vi "PvgeneratorOP500.vi"(8 "errin":errorcluster, 10 "network":path, 11 "path in":path) -> (0 "sortie d'erreur":errorcluster caption="errout", 1 "network out":path, 2 "tout bon":bool, 3 "Chaîne":string)   [LabVIEW 2020]
uses:
  VG/IS30%.vi
  VG/VG_OCV30min.vi
  VG/VG_OCV30max.vi
  VG/VG_OCV70min.vi
  VG/VG_OCV70max.vi
  VG/VG_OP400.vi
  VG/VG_ISOmin.vi
  VG/VG_DCIRmax.vi
  VG/VG_DCIRmin.vi
  VG/VG_DCIR+OUIouNON.vi
panel:
  out "nombre de remplacements":i32
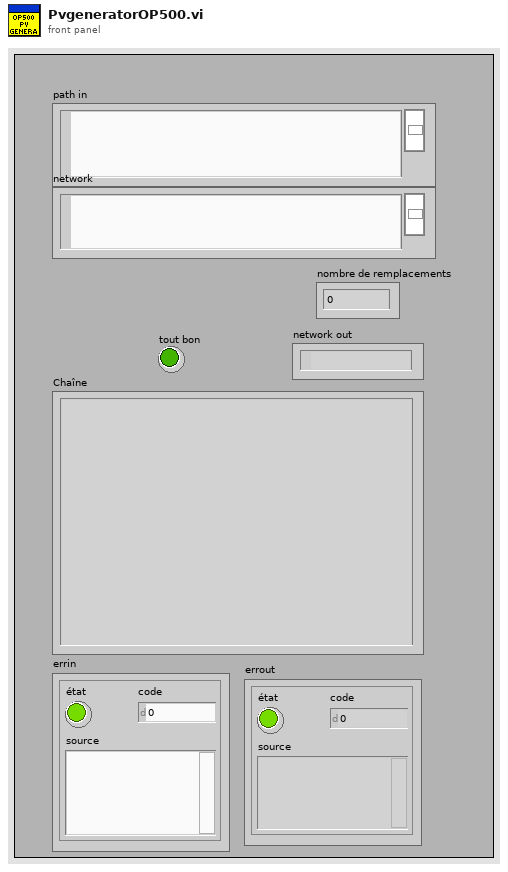
[diagram p1: front panel]
types:
  T1 = enum16{"open", "replace", "create", "open or create", "replace or create", "replace or create with confirmation"}
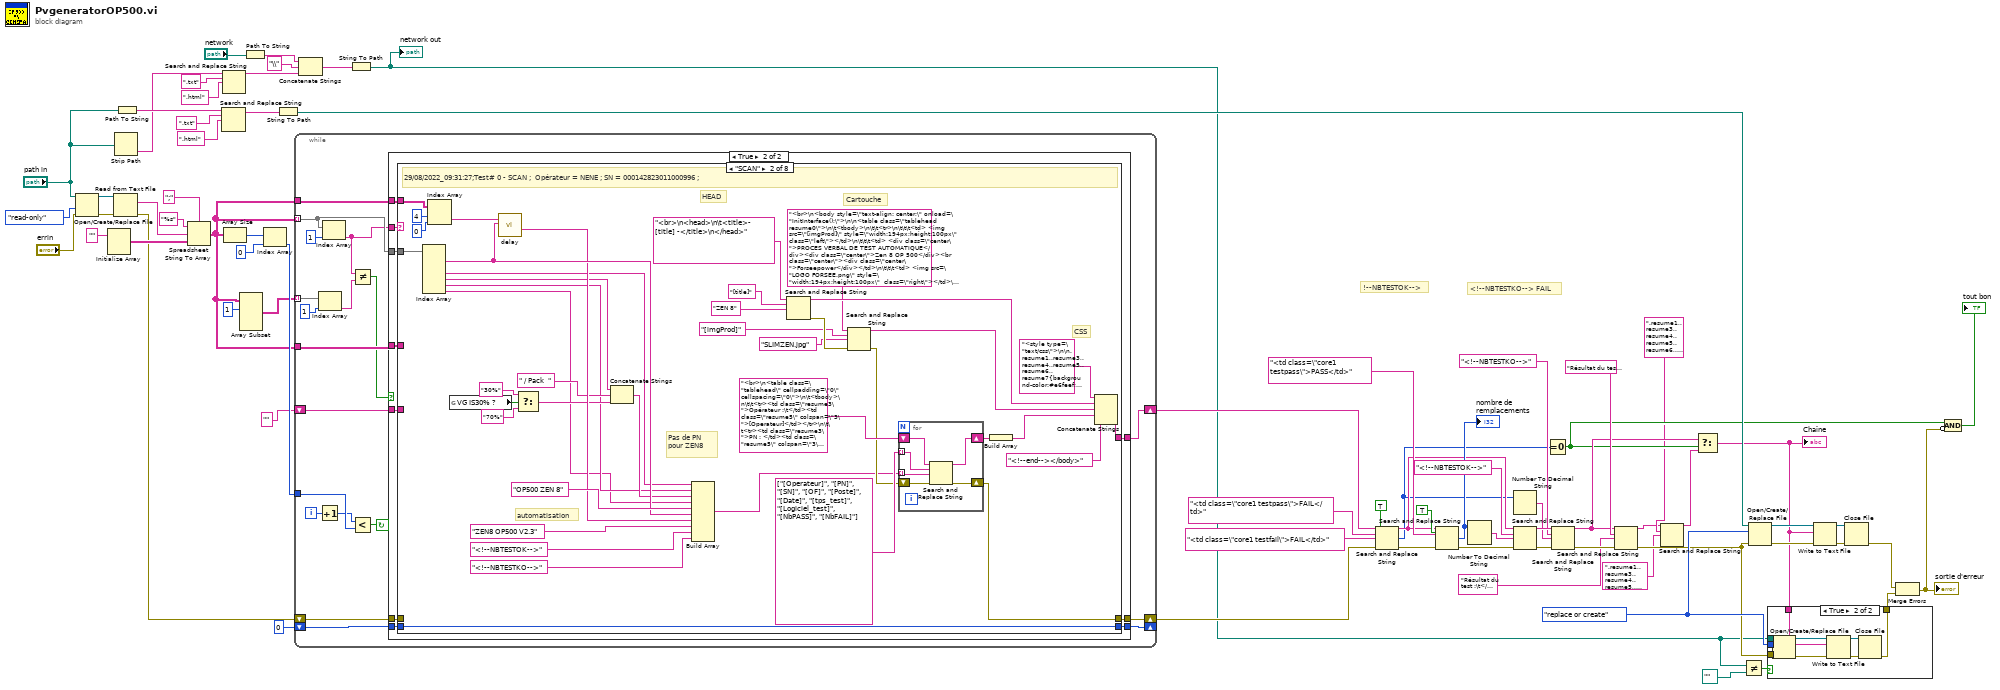
[diagram p0: block diagram]
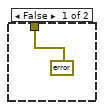
[diagram p2: hidden frame]
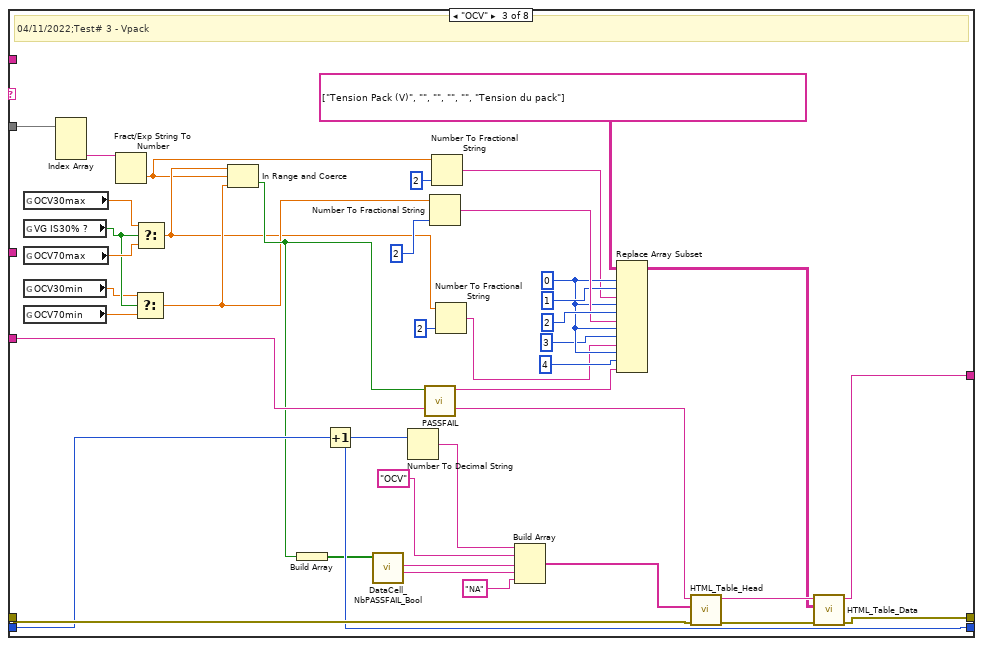
[diagram p5: hidden frame]
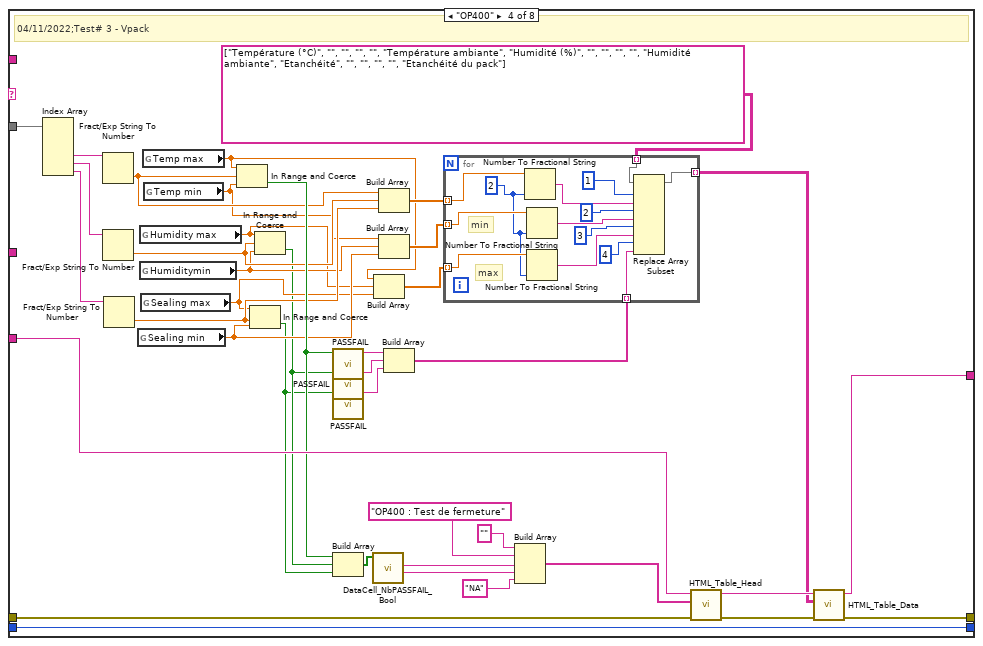
[diagram p6: hidden frame]
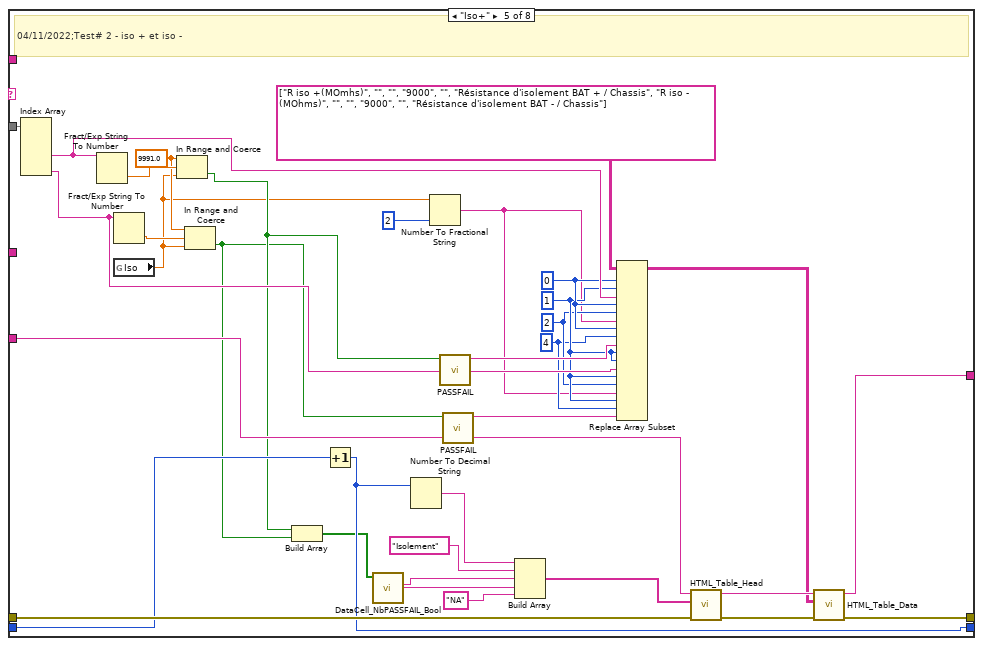
[diagram p7: hidden frame]
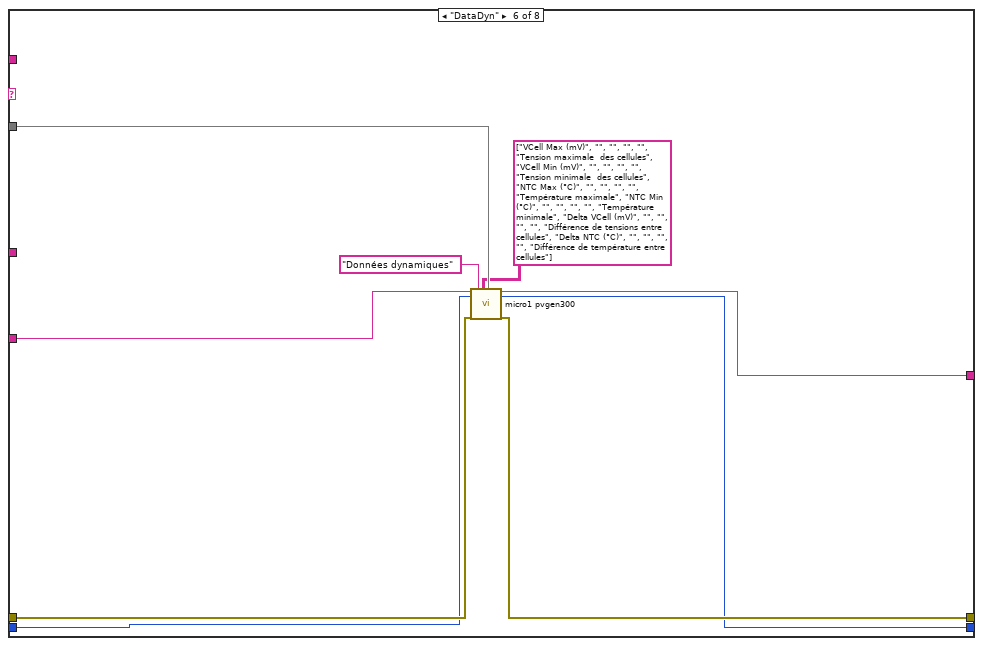
[diagram p8: hidden frame]
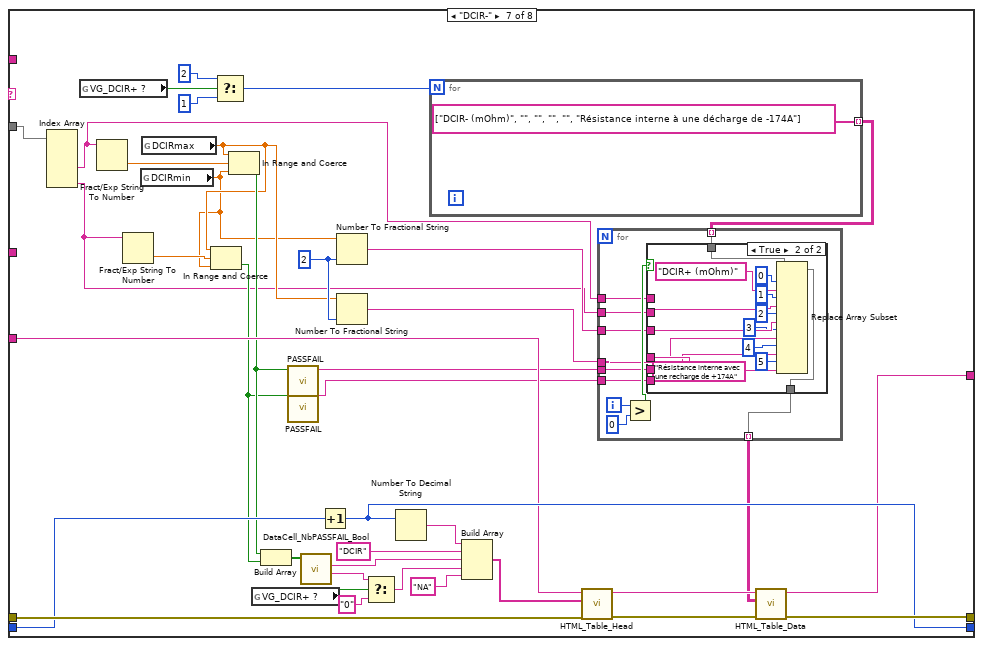
[diagram p9: hidden frame]
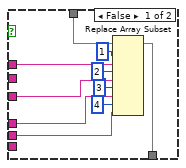
[diagram p10: hidden frame]
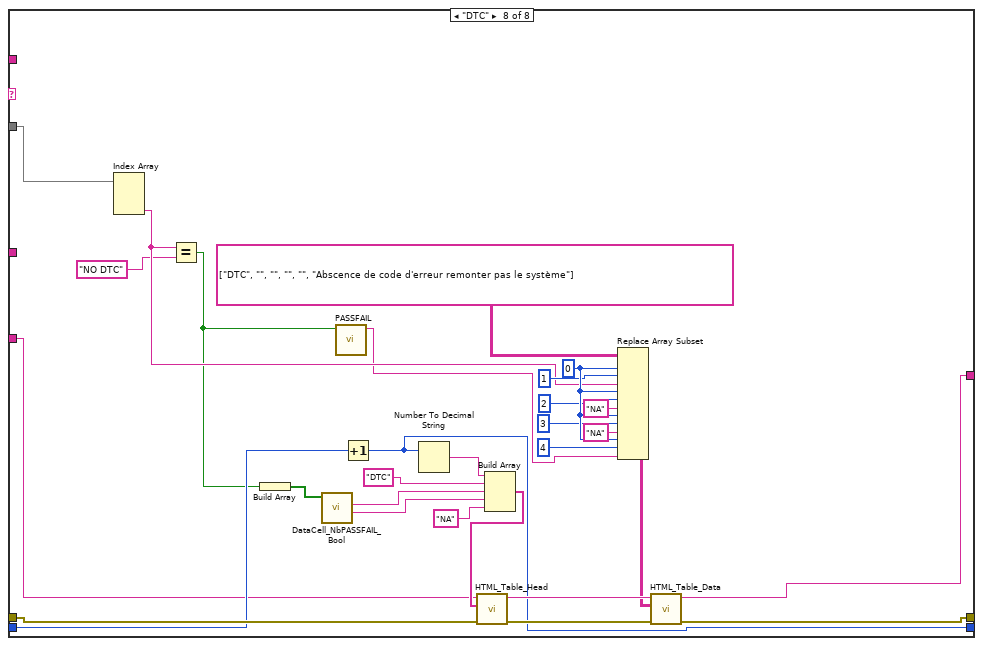
[diagram p11: hidden frame]
diagram:
  w32 = T1."replace or create" ("opération (0 : open)")
  # "<!--NBTESTKO--> FAIL"
  # "!--NBTESTOK-->"
  n1 = Open/Create/Replace File(file path (use dialog)="path in", error in="errin", access (0:read/write)=enum16{"read/write", "read-only", "write-only"}."read-only" ("accès (0 : read/write)")) -> (refnum out=w55:refnum<file>, error out=w72:errorcluster)  [unwired: 3 in, 1 out]
  n2 = Initialize Array("") -> (w70:string[][])  [unwired: 2 in]
  n3 = Read from Text File(file (use dialog)=w55, error in=w72) -> (text=w68:string, error out=w60:errorcluster)  [unwired: 2 in, 2 out]
  n4 = Strip Path(path="path in") -> (name=w13:string)  [unwired: 1 out]
  n5 = Path To String(path="path in") -> (string=w54:string)
  n6 = Spreadsheet String To Array(delimiter (Tab)=";" ("séparateur (Tabulation)"), format string="%s" ("chaîne de format"), spreadsheet string=w68, array type (2D Dbl)=w70) -> (array=w3:string[][])
  n7 = Search and Replace String(input string=w54, search string=".txt" ("chaîne recherchée"), replace string=".html" ("chaîne de remplacement (\"\")")) -> (result string=w51:string)  [unwired: 5 in, 3 out]
  n8 = Search and Replace String(input string=w13, search string=".txt" ("chaîne recherchée"), replace string=".html" ("chaîne de remplacement (\"\")")) -> (result string=w10:string)  [unwired: 5 in, 3 out]
  n9 = Array Size(array=w3) -> (size(s)=w66:i32[])
  n10 = Array Subset(array=w3, index (row)=1 ("indice")) -> (w1:string[][])  [unwired: 3 in]
  n11 = Path To String(path="network") -> (string=w12:string)
  n12 = Index Array(array=w66, index=0 ("indice")) -> (element=w64:i32)
  n13 = String To Path(string=w51) -> (path=w50:path)
  n14 = while {
    tunnel: w64 -> [w91]
    tunnel: w3 -> [w88] mode=indexing
    shift-right: [w87] -> w47
    shift-left: w60 -> [w86]
    shift-right: [w80] -> w49
    shift-left: "" -> [w85]
    shift-right: [w83] -> _
    shift-left: 0 -> [w84]
    tunnel: w3 -> [w82]
    tunnel: w3 -> [w79]
    tunnel: w1 -> [w77] mode=indexing
    i -> [w92]
    stop <- w90 continue-if-true
    n15 = Index Array(array=w77, index=1 ("indice")) -> (element=w76:string)
    n16 = Increment(x=w92) -> (x+1=w81:i32)
    n17 = Index Array(array=w88, index=1 ("indice")) -> (element=w75:string)
    n18 = Less?(x=w81, y=w91) -> (x < y?=w90:bool)
    n19 = Not Equal?(x=w75, y=w76) -> (x != y?=w74:bool)
    n20 = case shown="True" w74 {
      tunnel: w88 -> [_ w105]
      tunnel: [w94 w104] -> w87
      tunnel: w86 -> [w94 w103]
      tunnel: w85 -> [w95 w102]
      tunnel: w84 -> [w93 w101]
      tunnel: [w93 w100] -> w83
      tunnel: w82 -> [_ w99]
      tunnel: [w95 w98] -> w80
      tunnel: w75 -> [_ w97]
      tunnel: w79 -> [_ w96]
      frame False {
      }
      frame True {
        n21 = case shown="\"SCAN\"" w97 {
          tunnel: w103 -> [w108 _ w187 w227 w274 w291 w324 w391]
          tunnel: w105 -> [_ w149 w188 w228 w275 w287 w328 w381]
          tunnel: [w108 w128 w186 w226 w273 w290 w326 w392] -> w104
          tunnel: w102 -> [w106 _ w185 w225 w272 w285 w318 w382]
          tunnel: w101 -> [w107 w127 w184 w216 w271 w284 w323 w384]
          tunnel: [w107 w127 w183 w216 w270 w283 w320 w366] -> w100
          tunnel: w99 -> [_ _ _ _ _ _ _ _]
          tunnel: [w106 w126 w182 w224 w269 w289 w311 w380] -> w98
          tunnel: w96 -> [_ w125 _ _ _ _ _ _]
          frame "NULL", Default {
            # "NULL"
          }
          frame "SCAN" {
            # "automatisation"
            # "Pas de PN pour ZEN8"
            # "Cartouche"
            # "HEAD"
            # "CSS"
            # "29/08/2022_09:31:27;Test# 0 - SCAN ;  Opérateur = NENE ; SN = 000142823011000996 ;"
            n22 = Index Array(array=w149) -> (element #1=w121:string, element #3=w112:string, element #4=w111:string, element #5=w110:string, element #6=w109:string)  [unwired: 6 in, 1 out]
            n23 = Index Array(array=w125, index (row)=4, index (col)=0 ("disabled index (col)")) -> (element=w122:string)
            n24 = global read "IS30%.vi" "VG IS30% ?"() -> (w113:bool)
            n25 = call "delay.vi"("String"=w121, "String 2"=w122) -> ("Delay calculé"=w120:string)  [unwired: 9 in]
            n26 = Select(t="30%" ("y"), s=w113, f="70%" ("y")) -> (s? t:f=w116:string)
            n27 = Concatenate Strings(w111, " / Pack  " ("chaîne"), w116) -> (w118:string)
            n28 = Build Array(w112, w110, w118, w109, "OP500 ZEN 8" ("chaîne"), w121, w120, "ZEN8 OP500 V2.3" ("chaîne"), "<!--NBTESTOK-->" ("chaîne"), "<!--NBTESTKO-->" ("chaîne")) -> (w129:string[])
            n29 = Search and Replace String(input string="<br>\n<head>\n\t<title>- [title] -</title>\n</head>", search string="[title]" ("chaîne recherchée"), replace string="ZEN 8" ("Title")) -> (result string=w145:string, error out=w144:errorcluster)  [unwired: 5 in, 2 out]
            n30 = Search and Replace String(input string="<br>\n<body style=\"text-align: center;\" onload=\"InitInterface();\">\n\n<table class=\"tablehead resume0\">\n\t<tbody>\n\t\t<tr>\n\t\t\t<td> <img src=\"[imgProd]\" style=\"width:194px;height:100px\" class=\"left\"></td>\n\t\t\t<td> <div class=\"center\">PROCES VERBAL DE TEST AUTOMATIQUE</div><div class=\"center\">Zen 8 OP 500</div><br class=\"center\"><div class=\"center\">Forseepower</div></td>\n\t\t\t<td> <img src=\"LOGO FORSEE.png\" style=\"width:194px;height:100px\"  class=\"right\"></td>\n\t\t</tr>\n\t</tbody>\n</table>", search string="[imgProd]", replace string="SLIMZEN.jpg" ("imgProd"), error in=w144) -> (result string=w142:string, error out=w139:errorcluster)  [unwired: 4 in, 2 out]
            n31 = for {
              shift-right: [w154] -> w138
              shift-left: "<br>\n<table class=\"tablehead\" cellpadding=\"0\" cellspacing=\"0\">\n\t<tbody>\n\t\t<tr><td class=\"resume3\">Opérateur :\t</td><td class=\"resume5\" colspan=\"3\">[Operateur]</td></tr>\n\t\t<tr><td class=\"resume3\">PN : </td><td class=\"resume5\" colspan=\"3\">[PN]</td></tr>\n\t\t<tr><td class=\"resume3\">SN : </td><td class=\"resume5\" colspan=\"3\">[SN]</td></tr>\n\t\t<tr><td class=\"resume3\">OF : </td><td class=\"resume5\" colspan=\"3\">[OF]</td></tr>\n\t\t<tr><td class=\"resume3\">Poste : </td><td class=\"resume5\" colspan=\"3\">[Poste]</td></tr>\t\t\n\t\t<tr><td class=\"resume3\">Date du test : </td><td class=\"resume5\" colspan=\"3\">[Date]</td></tr>\n\t\t<tr><td class=\"resume3\">Temps de test : </td><td class=\"resume5\" colspan=\"3\">[tps_test]</td></tr>\n\t\t<tr><td class=\"resume3\">Logiciel de test :\t</td><td class=\"resume5\" colspan=\"3\">[Logiciel_test]</td></tr>\n\t\t<tr><td class=\"resume3\">Résultat du test :\t</td><td class=\"resume5\" colspan=\"3\"><div><span style=\"float:left\" id=\"result\"><font size = \"5pt\" color=\"green\"><b>CONFORME</b></font><b><font size = \"5pt\"> ( </font><font size = \"5pt\" color=\"green\">[NbPASS] PASS </font>  <font size = \"5pt\"> / </font><font size = \"5pt\" color=\"red\">[NbFAIL] FAIL</font> <font size = \"5pt\"> ) </font></b></span></div></td></tr>\n\t</tbody>\n</table>" -> [w155]
              tunnel: string[] ["[Operateur]", "[PN]", "[SN]", "[OF]", "[Poste]", "[Date]", "[tps_test]", "[Logiciel_test]", "[NbPASS]", "[NbFAIL]"] -> [w151] mode=indexing
              tunnel: w129 -> [w150] mode=indexing
              shift-right: [w152] -> w128
              shift-left: w139 -> [w153]
              n32 = Search and Replace String(input string=w155, search string=w151, replace string=w150, error in=w153) -> (result string=w154:string, error out=w152:errorcluster)  [unwired: 4 in, 2 out]
            }
            n33 = Build Array(w138) -> (w137:string[])
            n34 = Concatenate Strings("<style type=\"text/css\">\n\n.resume1,.resume3,.resume4,.resume5,.resume6,.resume7{background-color:#e6feef;padding:7px;border:1px solid black;}\n.resume0{border:1px solid black;background-color:#e6feef;font-weight: bold;padding:0px;text-align: center;}\n.resume1{width:350px;text-align:right;font-weight:bold;}\n.resume3{width:350px;text-align:right;border-top:0px solid black;font-weight:bold;}\n.resume4{border-left:0px solid black;width:290px;}\n.resume5{width:290px;border-left:0px solid black;border-top:0px solid black;}\n.resume6{border-left:0px solid black;width:60px;}\n.resume7{border-left:0px solid black;border-top:0px solid black;width:60px;}\n.title1{text-align: left;background-color:#e6f4fe;padding:10px;border:1px solid #101010;}\n.title2{width: 30px;text-align: center;background-color:#e6f4fe;padding:1px;border:1px solid #101010;border-left:0px solid black;font-weight: bold;}\n.title2 a:link{text-decoration:none;}\n.entete0,.entete1,.entete2,.time2{text-align: center;background-color:#feeec9;padding:7px;border:1px solid black;font-weight: bold;}\n.entete0{width:45px;border-right:0px solid black;}\n.entete1{width:505px;}\n.entete2{width:95px;border-right:0px solid black;}\n.time2{border-left:0px solid black;width:145px;font-size:11px;}\n.core0,.core1,.core2,.core3,.core4,.time{text-align: center;background-color:#fafed3;padding:7px;border:1px solid black;}\n.core0, .core1,.core3,.core4{width:95px;border-top:0px solid black;border-right:0px solid black;}\n.core0{width:45px;}\n.core2{border-top:0px solid black;width:505px;}\n.core3{width:200px;}\n.core4{width:300px;}\n.time{width:145px;border-top:0px solid black;border-left:0px solid black;font-size:11px;}\n.false .core0,.false .core1,.false .core2,.false .core3,.false .core4,.false .time{background-color:#f4f4f4;}\n.false .entete0,.false .entete1,.false .entete2,.false .time2{background-color:#dadada;}\n.false .title1,.false .title2,.false .resultentete .testpass,.false .resultentete .testfail,.false .resultentete .testtime{background-color:#c5cac9;color: blue;}\n.false .title2 a:link{text-decoration:none;color: blue;}\n.comment1,.comment2,.time3{width: 890px;background-color:#e9e8e9;padding:7px;border:1px solid black;border-top:0px solid black;text-align:left;}\n.comment2{border-right:0px solid black;width: 45px;text-align: center;}\n.time3{width: 145px;border-left:0px solid black;font-size:11px;}\n.fixe1{background: -moz-linear-gradient(center top , #101010 10%, #555555 80%) repeat scroll 0 0 transparent;background: -webkit-gradient(linear, left top, left bottom, from(#101010), to(#555555));border:2px solid orange;position : fixed;margin-top:20px;display:none;overflow-y:scroll;max-height:350px;text-shadow: 0px 0px 0 #333333;text-align:left;font-size:10px;padding:10px;margin-left:-162px;border-radius: 15px 15px 15px 15px;}\n.menufixe, .menufixelock{background: -moz-linear-gradient(center top , #101010 80%, transparent 20%) repeat scroll 0 0 transparent;background: -webkit-gradient(linear, left top, left bottom, from(#101010), color-stop(0.65, #101010), to(transparent)) repeat scroll 0 0 transparent;margin: -52px 0px 0px -9px;width:100%;position:fixed;height:55px;-moz-transition: margin 1s;-webkit-transition: margin 1s;}\n.menufixelock, .menufixe:hover{margin: -9px 0px 0px -9px;}\n.lockmenu, .separation,.separationmenu{text-align:center;background: -moz-linear-gradient(center top , #555555 10%, #111111 80%) repeat scroll 0 0 transparent;background: -webkit-gradient(linear, left top, left bottom, from(#555555), to(#111111));border: 1px solid white;border-radius: 10px 10px 10px 10px;box-shadow: 0 -1px 1px #555555 inset;color: #999999;font-weight: bold;width: 100px;padding: 2px;text-decoration: none;}\n.tablehead{width: 1000px;font-family: Verdana;font-size: 12px;margin-left: auto;margin-right: auto;}\n.tablenull{font-family: Verdana;font-size: 11px;margin-left: auto;margin-right: auto;}\n.separationmenu:hover div{display: inline;}\n.lockmenu:hover, .separation:hover,.separationmenu:hover{border: 1px solid orange;cursor:pointer;}\n.lockmenu:hover{border: 1px solid red;cursor:pointer;}\n.separationright{padding:10px;}\ndiv a:link{text-decoration:none;color:#cbcbcb;}\ndiv a:hover{text-decoration:underline;color:#cbcbcb;}\nspan a:link{text-decoration:none;color:#cbcbcb;}\nspan a:hover{text-decoration:none;color:#cbcbcb;}\n.false{color: blue;}\n.testpass{color: green;font-weight: bold;}\n.testfail{color: red;font-weight: bold;}\n.testtime{color: blue;font-weight: bold;}\n.resultentete{font-weight: bold;font-size: 11px;min-width: 200px;text-align:right;}\n.infohard{border: 1px solid black;background-color: white;text-align: center;width: 16px;height: 16px;border-radius: 5px;font-weight: bold;box-shadow: 0 -1px 2px #555555 inset;}\n.infohard:hover{background-color:#feeec9;cursor:pointer;}\n.footerhard{padding-top:30px;}\n.confighard{font-size:10px;width:110px;}\n.circlemain{margin-left:auto;margin-right:auto;}\n.circletext,.circleform{padding-top: 3px;text-align:center;font-size: 10px;width:200px;}\n.circleform{padding-bottom: 3px;padding-top: 1px;}\n.circle{border: 1px solid black;border-collapse: collapse;border-radius: 15px;box-shadow: 1px 1px 0 #505050;height: 15px;width: 15px;display:inline-block;}\n.bookmarkon, .bookmarkoff{background-color: yellow;border: 1px solid black;border-collapse: collapse;border-radius: 10px 10px 10px 10px;box-shadow: 1px 1px 0 #505050;height: 12px;width: 12px;position: absolute;margin-left:22px;cursor: help;}\n.bookmarkoff{background-color: transparent;border: 1px solid #CECECE;box-shadow: none;cursor: copy;}\n.false .bookmarkoff{background-color: transparent;border: 1px solid #E6E1E1;box-shadow: none;cursor: copy;}\n.bookmarkmaster{height: 15px;margin-right: 12px;width: 60px;}\n.bookmarkmaster:hover .bookmarkprev,.bookmarkmaster:hover .bookmarksuiv{display:block;}\n.bookmarkprev, .bookmarksuiv {cursor: pointer;font-size: 25px;font-weight: bold;margin-top: -10px;position: absolute;display:none;}\n.bookmarkprev{margin-left: 2px;}\n.bookmarksuiv{margin-left: 43px;}\n.plus, .moins{background-color: #F4F4F4;border: 1px solid #848484;border-radius: 20px;color: #848484;font-family: arial;font-size: 16px;font-weight: bold;height: 20px;margin-left: 4px;text-align: center;width: 20px;}\n.moins{font-size: 15px;}\n.plus:hover, .moins:hover{background-color: #DADADA;border: 1px solid black;color: black;cursor:pointer;}\n.backtothetop {position: fixed; right: 50%; margin-right: -555px; bottom: 10px; font-size: 35px; font-weight: bold; border: 1px solid #7D7B91; width: 40px; height: 40px; line-height:52px; text-align: center;border-radius: 8px; opacity: 0.25; background-color: #F5F5F5; color:#7D7B91;}\n.backtothetop:hover {opacity: 1; cursor:pointer;}\n.libversion {font-size: 8px;font-weight: normal;padding-right: 10px;text-align: right;}\n.lockmenu {width: 18px;font-size: 12px;}\n.left {display: block; margin-left: 1px;margin-right: auto;}\n.right {display: block; margin-right: 1px;margin-left: auto;}\n.center {display: block; margin-left: auto;margin-right: auto;}\n\n</style>", w145, w142, w137, "<!--end--></body>") -> (w126:string)
          }
          frame "OCV" {
            w170 = 0 ("index (row)")
            # "04/11/2022;Test# 3 - Vpack"
            n35 = global read "VG_OCV30max.vi" "OCV30max"() -> (w165:dbl)
            n36 = global read "IS30%.vi" "VG IS30% ?"() -> (w163:bool)
            n37 = global read "VG_OCV70max.vi" "OCV70max"() -> (w164:dbl)
            n38 = global read "VG_OCV30min.vi" "OCV30min"() -> (w162:dbl)
            n39 = global read "VG_OCV70min.vi" "OCV70min"() -> (w161:dbl)
            n40 = Index Array(array=w188) -> (element #3=w173:string)  [unwired: 3 in, 2 out]
            n41 = Fract/Exp String To Number(string=w173) -> (number=w158:dbl)  [unwired: 3 in, 1 out]
            n42 = Select(t=w162, s=w163, f=w161) -> (s? t:f=w160:dbl)
            n43 = Select(t=w165, s=w163, f=w164) -> (s? t:f=w159:dbl)
            n44 = In Range and Coerce(upper limit=w159, x=w158, lower limit=w160) -> (In Range?=w168:bool)  [unwired: 1 out]
            n45 = Build Array(w168) -> (w180:bool[])
            n46 = Increment(x=w184) -> (x+1=w183:i32)
            n47 = call <userlib>:"DataCell_NbPASSFAIL_Bool.vi"("Tableau en entrée"=w180) -> ("Chaîne"=w178:string, "Chaîne 2"=w179:string)  [unwired: 8 in, 1 out]
            n48 = Number To Decimal String(number=w183) -> (decimal integer string=w191:string)  [unwired: 1 in]
            n49 = call <userlib>:"PASSFAIL.vi"("E"=w168) -> ("S"=w172:string)  [unwired: 10 in]
            n50 = Number To Fractional String(number=w160, precision (6)=i16 2) -> (F-format string=w176:string)  [unwired: 2 in]
            n51 = Number To Fractional String(number=w158, precision (6)=i16 2 ("précision (6)")) -> (F-format string=w157:string)  [unwired: 2 in]
            n52 = Number To Fractional String(number=w159, precision (6)=i16 2) -> (F-format string=w166:string)  [unwired: 2 in]
            n53 = Build Array(w191, "OCV" ("élément"), w179, w178, "NA" ("élément")) -> (w194:string[])
            n54 = Replace Array Subset(array=string[][] [["Tension Pack (V)", "", "", "", "", "Tension du pack"]] ("Tableau"), new element #1=w157, index (row) #1=w170, index (col) #1=1 ("disabled index (col)"), new element #2=w176, index (row) #2=w170, index (col) #2=2 ("disabled index (col)"), new element #3=w166, index (row) #3=w170, index (col) #3=3 ("disabled index (col)"), new element #4=w172, index (row) #4=w170, index (col) #4=4 ("disabled index (col)")) -> (w181:string[][])
            n55 = call "HTML_Table_Head.vi"("entrée d'erreur (pas d'erreur)"=w187, "Tableau"=w194, "chaîne en entrée"=w185) -> ("sortie d'erreur"=w193:errorcluster, "result string"=w192:string)  [unwired: 7 in]
            n56 = call "HTML_Table_Data.vi"("entrée d'erreur (pas d'erreur)"=w193, "Tableau"=w181, "chaîne en entrée"=w192) -> ("sortie d'erreur"=w186:errorcluster, "result string"=w182:string)  [unwired: 7 in]
          }
          frame "OP400" {
            # "04/11/2022;Test# 3 - Vpack"
            n57 = Index Array(array=w228) -> (element #3=w219:string, element #4=w215:string, element #5=w214:string)  [unwired: 5 in, 2 out]
            n58 = Fract/Exp String To Number(string=w219) -> (number=w213:dbl)  [unwired: 3 in, 1 out]
            n59 = Fract/Exp String To Number(string=w215) -> (number=w212:dbl)  [unwired: 3 in, 1 out]
            n60 = Fract/Exp String To Number(string=w214) -> (number=w211:dbl)  [unwired: 3 in, 1 out]
            n61 = global read "VG_OP400.vi" "Sealing min"() -> (w207:dbl)
            n62 = global read "VG_OP400.vi" "Humidity max"() -> (w204:dbl)
            n63 = global read "VG_OP400.vi" "Humiditymin"() -> (w208:dbl)
            n64 = global read "VG_OP400.vi" "Sealing max"() -> (w203:dbl)
            n65 = global read "VG_OP400.vi" "Temp max"() -> (w205:dbl)
            n66 = global read "VG_OP400.vi" "Temp min"() -> (w209:dbl)
            n67 = In Range and Coerce(upper limit=w205, x=w213, lower limit=w209) -> (In Range?=w218:bool)  [unwired: 1 out]
            n68 = In Range and Coerce(upper limit=w203, x=w211, lower limit=w207) -> (In Range?=w199:bool)  [unwired: 1 out]
            n69 = In Range and Coerce(upper limit=w204, x=w212, lower limit=w208) -> (In Range?=w200:bool)  [unwired: 1 out]
            n70 = call <userlib>:"PASSFAIL.vi"("E"=w218) -> ("S"=w201:string)  [unwired: 10 in]
            n71 = call <userlib>:"PASSFAIL.vi"("E"=w200) -> ("S"=w198:string)  [unwired: 10 in]
            n72 = call <userlib>:"PASSFAIL.vi"("E"=w199) -> ("S"=w197:string)  [unwired: 10 in]
            n73 = Build Array(w218, w200, w199) -> (w222:bool[])
            n74 = call <userlib>:"DataCell_NbPASSFAIL_Bool.vi"("Tableau en entrée"=w222) -> ("Chaîne"=w220:string, "Chaîne 2"=w221:string)  [unwired: 8 in, 1 out]
            n75 = Build Array(w205, w204, w203) -> (w202:dbl[])
            n76 = Build Array(w213, w212, w211) -> (w210:dbl[])
            n77 = Build Array(w209, w208, w207) -> (w206:dbl[])
            n78 = Build Array(w201, w198, w197) -> (w196:string[])
            n79 = for {
              tunnel: string[][] [["Température (°C)", "", "", "", "", "Température ambiante"], ["Humidité (%)", "", "", "", "", "Humidité ambiante"], ["Etanchéité", "", "", "", "", "Etanchéité du pack"]] ("Tableau") -> [w248] mode=indexing
              tunnel: [w244] -> w223 mode=indexing
              tunnel: w210 -> [w243] mode=indexing
              tunnel: w206 -> [w240] mode=indexing
              tunnel: w202 -> [w239] mode=indexing
              tunnel: w196 -> [w235] mode=indexing
              w238 = i16 2 ("précision (6)")
              # "max"
              # "min"
              n80 = Number To Fractional String(number=w243, precision (6)=w238) -> (F-format string=w245:string)  [unwired: 2 in]
              n81 = Number To Fractional String(number=w240, precision (6)=w238) -> (F-format string=w246:string)  [unwired: 2 in]
              n82 = Number To Fractional String(number=w239, precision (6)=w238) -> (F-format string=w237:string)  [unwired: 2 in]
              n83 = Replace Array Subset(array=w248, new element #1=w245, index #1=1 ("index"), new element #2=w246, index #2=2 ("index"), new element #3=w237, index #3=3 ("index"), new element #4=w235, index #4=4 ("index")) -> (w244:string[])
            }
            n84 = Build Array("" ("element"), "OP400 : Test de fermeture" ("élément"), w221, w220, "NA" ("élément")) -> (w233:string[])
            n85 = call "HTML_Table_Head.vi"("entrée d'erreur (pas d'erreur)"=w227, "Tableau"=w233, "chaîne en entrée"=w225) -> ("sortie d'erreur"=w232:errorcluster, "result string"=w231:string)  [unwired: 7 in]
            n86 = call "HTML_Table_Data.vi"("entrée d'erreur (pas d'erreur)"=w232, "Tableau"=w223, "chaîne en entrée"=w231) -> ("sortie d'erreur"=w226:errorcluster, "result string"=w224:string)  [unwired: 7 in]
          }
          frame "Iso+" {
            w250 = 9991.0 ("limite supérieure")
            w257 = 4 ("disabled index (col)")
            w258 = 2 ("disabled index (col)")
            w259 = 1 ("disabled index (col)")
            w262 = 0 ("index (row)")
            # "04/11/2022;Test# 2 - iso + et iso -"
            n87 = Index Array(array=w275) -> (element #3=w263:string, element #5=w260:string)  [unwired: 5 in, 3 out]
            n88 = Fract/Exp String To Number(string=w263) -> (number=w254:dbl)  [unwired: 3 in, 1 out]
            n89 = Fract/Exp String To Number(string=w260) -> (number=w251:dbl)  [unwired: 3 in, 1 out]
            n90 = global read "VG_ISOmin.vi" "Iso"() -> (w249:dbl)
            n91 = In Range and Coerce(upper limit=w250, x=w254, lower limit=w249) -> (In Range?=w253:bool)  [unwired: 1 out]
            n92 = In Range and Coerce(upper limit=w250, x=w251, lower limit=w249) -> (In Range?=w252:bool)  [unwired: 1 out]
            n93 = Build Array(w253, w252) -> (w267:bool[])
            n94 = Increment(x=w271) -> (x+1=w270:i32)
            n95 = call <userlib>:"DataCell_NbPASSFAIL_Bool.vi"("Tableau en entrée"=w267) -> ("Chaîne"=w265:string, "Chaîne 2"=w266:string)  [unwired: 8 in, 1 out]
            n96 = Number To Decimal String(number=w270) -> (decimal integer string=w278:string)  [unwired: 1 in]
            n97 = Number To Fractional String(number=w249, precision (6)=i16 2) -> (F-format string=w256:string)  [unwired: 2 in]
            n98 = call <userlib>:"PASSFAIL.vi"("E"=w253) -> ("S"=w261:string)  [unwired: 10 in]
            n99 = call <userlib>:"PASSFAIL.vi"("E"=w252) -> ("S"=w255:string)  [unwired: 10 in]
            n100 = Build Array(w278, "Isolement" ("élément"), w266, w265, "NA" ("élément")) -> (w281:string[])
            n101 = Replace Array Subset(array=string[][] [["R iso +(MOmhs)", "", "", "9000", "", "Résistance d'isolement BAT + / Chassis"], ["R iso - (MOhms)", "", "", "9000", "", "Résistance d'isolement BAT - / Chassis"]] ("Tableau"), new element #1=w263, index (row) #1=w262, index (col) #1=w259, new element #2=w256, index (row) #2=w262, index (col) #2=w258, new element #3=w261, index (row) #3=w262, index (col) #3=w257, new element #4=w260, index (row) #4=w259, index (col) #4=w259, new element #5=w256, index (row) #5=w259, index (col) #5=w258, new element #6=w255, index (row) #6=w259, index (col) #6=w257) -> (w268:string[][])
            n102 = call "HTML_Table_Head.vi"("entrée d'erreur (pas d'erreur)"=w274, "Tableau"=w281, "chaîne en entrée"=w272) -> ("sortie d'erreur"=w280:errorcluster, "result string"=w279:string)  [unwired: 7 in]
            n103 = call "HTML_Table_Data.vi"("entrée d'erreur (pas d'erreur)"=w280, "Tableau"=w268, "chaîne en entrée"=w279) -> ("sortie d'erreur"=w273:errorcluster, "result string"=w269:string)  [unwired: 7 in]
          }
          frame "DataDyn" {
            n104 = call "micro1 pvgen300.vi"("FluxStrIn"=w285, "Numin"=w284, "errin"=w291, "Data label"="Données dynamiques" ("testlabel"), "tab ref"=string[][] [["VCell Max (mV)", "", "", "", "", "Tension maximale  des cellules"], ["VCell Min (mV)", "", "", "", "", "Tension minimale  des cellules"], ["NTC Max (°C)", "", "", "", "", "Température maximale"], ["NTC Min (°C)", "", "", "", "", "Température minimale"], ["Delta VCell (mV)", "", "", "", "", "Différence de tensions entre cellules"], ["Delta NTC (°C)", "", "", "", "", "Différence de température entre cellules"]] ("Tableau"), "ligne à traiter"=w287) -> ("result string"=w289:string, "Numout"=w283:i32, "errout"=w290:errorcluster)  [unwired: 11 in]
          }
          frame "DCIR-" {
            w308 = i16 2 ("précision (6)")
            n105 = Index Array(array=w328) -> (element #3=w314:string, element #5=w296:string)  [unwired: 5 in, 3 out]
            n106 = global read "VG_DCIR+OUIouNON.vi" "VG_DCIR+ ?"() -> (w303:bool)
            n107 = Fract/Exp String To Number(string=w314) -> (number=w325:dbl)  [unwired: 3 in, 1 out]
            n108 = Fract/Exp String To Number(string=w296) -> (number=w305:dbl)  [unwired: 3 in, 1 out]
            n109 = global read "VG_DCIRmin.vi" "DCIRmin"() -> (w298:dbl)
            n110 = global read "VG_DCIRmax.vi" "DCIRmax"() -> (w299:dbl)
            n111 = In Range and Coerce(upper limit=w299, x=w305, lower limit=w298) -> (In Range?=w304:bool)  [unwired: 1 out]
            n112 = Select(t=i16 2 ("précision (6)"), s=w303, f=i16 1) -> (s? t:f=w300:i16)
            n113 = In Range and Coerce(upper limit=w299, x=w325, lower limit=w298) -> (In Range?=w310:bool)  [unwired: 1 out]
            n114 = global read "VG_DCIR+OUIouNON.vi" "VG_DCIR+ ?"() -> (w295:bool)
            n115 = Build Array(w310, w304) -> (w317:bool[])
            n116 = call <userlib>:"PASSFAIL.vi"("E"=w310) -> ("S"=w309:string)  [unwired: 10 in]
            n117 = call <userlib>:"PASSFAIL.vi"("E"=w304) -> ("S"=w297:string)  [unwired: 10 in]
            n118 = call <userlib>:"DataCell_NbPASSFAIL_Bool.vi"("Tableau en entrée"=w317) -> ("Chaîne"=w294:string, "Chaîne 2"=w316:string)  [unwired: 8 in, 1 out]
            n119 = Increment(x=w323) -> (x+1=w320:i32)
            n120 = Number To Fractional String(number=w298, precision (6)=w308) -> (F-format string=w307:string)  [unwired: 2 in]
            n121 = Number To Fractional String(number=w299, precision (6)=w308) -> (F-format string=w306:string)  [unwired: 2 in]
            n122 = Select(t=w294, s=w295, f="0") -> (s? t:f=w293:string)
            n123 = Number To Decimal String(number=w320) -> (decimal integer string=w322:string)  [unwired: 1 in]
            n124 = for {
              N: w300 -> [_]
              tunnel: [string[] ["DCIR- (mOhm)", "", "", "", "", "Résistance interne à une décharge de -174A"] ("Tableau")] -> w329 mode=indexing
            }
            n125 = Build Array(w322, "DCIR" ("élément"), w316, w293, "NA" ("élément")) -> (w319:string[])
            n126 = call "HTML_Table_Head.vi"("entrée d'erreur (pas d'erreur)"=w324, "Tableau"=w319, "chaîne en entrée"=w318) -> ("sortie d'erreur"=w327:errorcluster, "result string"=w313:string)  [unwired: 7 in]
            n127 = for {
              tunnel: w329 -> [w340] mode=indexing
              tunnel: w314 -> [w335]
              tunnel: [w339] -> w312 mode=indexing
              tunnel: w309 -> [w332]
              tunnel: w307 -> [w334]
              tunnel: w306 -> [w333]
              tunnel: w296 -> [w331]
              tunnel: w297 -> [w330]
              i -> [w338]
              n128 = Greater?(x=w338, y=0) -> (0:w336:bool)
              n129 = case shown="True" w336 {
                tunnel: w340 -> [w350 w364]
                tunnel: [w349 w353] -> w339
                tunnel: w335 -> [w347 _]
                tunnel: w334 -> [w345 w358]
                tunnel: w333 -> [w343 w356]
                tunnel: w332 -> [w342 _]
                tunnel: w331 -> [_ w360]
                tunnel: w330 -> [_ w354]
                frame False {
                  n130 = Replace Array Subset(array=w350, new element #1=w347, index #1=1 ("index"), new element #2=w345, index #2=2 ("index"), new element #3=w343, index #3=3 ("index"), new element #4=w342, index #4=4 ("index")) -> (w349:string[])
                }
                frame True {
                  n131 = Replace Array Subset(array=w364, new element #1="DCIR+ (mOhm)" ("new element/subarray"), index #1=0 ("index"), new element #2=w360, index #2=1 ("index"), new element #3=w358, index #3=2 ("index"), new element #4=w356, index #4=3 ("index"), new element #5=w354, index #5=4 ("index"), new element #6="Résistance interne avec une recharge de +174A" ("new element/subarray"), index #6=5 ("index")) -> (w353:string[])
                }
              }
            }
            n132 = call "HTML_Table_Data.vi"("entrée d'erreur (pas d'erreur)"=w327, "Tableau"=w312, "chaîne en entrée"=w313) -> ("sortie d'erreur"=w326:errorcluster, "result string"=w311:string)  [unwired: 7 in]
          }
          frame "DTC" {
            w377 = 0 ("indice (ligne)")
            n133 = Index Array(array=w381) -> (element #3=w370:string)  [unwired: 3 in, 2 out]
            n134 = Equal?(x=w370, y="NO DTC") -> (x = y?=w369:bool)
            n135 = Build Array(w369) -> (w388:bool[])
            n136 = call <userlib>:"DataCell_NbPASSFAIL_Bool.vi"("Tableau en entrée"=w388) -> ("Chaîne"=w386:string, "Chaîne 2"=w387:string)  [unwired: 8 in, 1 out]
            n137 = call <userlib>:"PASSFAIL.vi"("E"=w369) -> ("S"=w368:string)  [unwired: 10 in]
            n138 = Increment(x=w384) -> (x+1=w366:i32)
            n139 = Number To Decimal String(number=w366) -> (decimal integer string=w390:string)  [unwired: 1 in]
            n140 = Build Array(w390, "DTC" ("élément"), w387, w386, "NA" ("élément")) -> (w383:string[])
            n141 = call "HTML_Table_Head.vi"("entrée d'erreur (pas d'erreur)"=w391, "Tableau"=w383, "chaîne en entrée"=w382) -> ("sortie d'erreur"=w394:errorcluster, "result string"=w393:string)  [unwired: 7 in]
            n142 = Replace Array Subset(array=string[][] [["DTC", "", "", "", "", "Abscence de code d'erreur remonter pas le système"]] ("Tableau"), new element #1=w370, index (row) #1=w377, index (col) #1=1 ("indice désactivé (col)"), new element #2="NA" ("nouvel élément/sous-tableau"), index (row) #2=w377, index (col) #2=2 ("indice désactivé (col)"), new element #3="NA" ("nouvel élément/sous-tableau"), index (row) #3=w377, index (col) #3=3 ("indice désactivé (col)"), new element #4=w368, index (row) #4=w377, index (col) #4=4 ("indice désactivé (col)")) -> (w379:string[][])
            n143 = call "HTML_Table_Data.vi"("entrée d'erreur (pas d'erreur)"=w394, "Tableau"=w379, "chaîne en entrée"=w393) -> ("sortie d'erreur"=w392:errorcluster, "result string"=w380:string)  [unwired: 7 in]
          }
        }
      }
    }
  }
  n144 = Concatenate Strings(w12, "\\" ("chaîne"), w10) -> (w9:string)
  n145 = String To Path(string=w9) -> (path=w15:path)
  "network out" <- w15
  n146 = Search and Replace String(replace all?=TRUE ("tout remplacer ? (F)"), input string=w49, search string="<td class=\"core1 testpass\">FAIL</td>" ("chaîne recherchée"), replace string="<td class=\"core1 testfail\">FAIL</td>" ("chaîne de remplacement (\"\")"), error in=w47) -> (result string=w33:string, number of replacements=w28:i32, error out=w44:errorcluster)  [unwired: 3 in, 1 out]
  n147 = Search and Replace String(replace all?=TRUE ("tout remplacer ? (F)"), input string=w33, search string="<td class=\"core1 testpass\">PASS</td>" ("chaîne recherchée"), error in=w44) -> (number of replacements=w36:i32, error out=w40:errorcluster)  [unwired: 4 in, 2 out]
  "nombre de remplacements" <- w36
  n148 = Number To Decimal String(number=w36) -> (decimal integer string=w35:string)  [unwired: 1 in]
  n149 = Number To Decimal String(number=w28) -> (decimal integer string=w34:string)  [unwired: 1 in]
  n150 = Search and Replace String(input string=w33, search string="<!--NBTESTOK-->" ("chaîne recherchée"), replace string=w35, error in=w40) -> (result string=w41:string, error out=w39:errorcluster)  [unwired: 4 in, 2 out]
  n151 = Equal To 0?(x=w28) -> (x = 0?=w20:bool)
  n152 = Search and Replace String(input string=w41, search string="<!--NBTESTKO-->" ("chaîne recherchée"), replace string=w34, error in=w39) -> (result string=w23:string, error out=w27:errorcluster)  [unwired: 4 in, 2 out]
  n153 = Search and Replace String(input string=w23, search string="Résultat du test :\t</td><td class=\"resume5\" colspan=\"3\"><div><span style=\"float:left\" id=\"result\"><font size = \"5pt\" color=\"green\"><b>CONFORME</b>", replace string="Résultat du test :\t</td><td class=\"resume5\" colspan=\"3\"><div><span style=\"float:left\" id=\"result\"><font  size = \"5pt\" color=\"red\"><b>NON CONFORME</b>", error in=w27) -> (result string=w5:string, error out=w26:errorcluster)  [unwired: 4 in, 2 out]
  n154 = Search and Replace String(input string=w5, search string=".resume1,.resume3,.resume4,.resume5,.resume6,.resume7{background-color:#e6feef;padding:7px;border:1px solid black;}\n.resume0{border:1px solid black;background-color:#e6feef;font-weight: bold;padding:0px;text-align: center;}", replace string=".resume1,.resume3,.resume4,.resume5,.resume6,.resume7{background-color:#fdebd0;padding:7px;border:1px solid black;}\n.resume0{border:1px solid black;background-color:#fdebd0;font-weight: bold;padding:0px;text-align: center;}") -> (result string=w4:string)  [unwired: 5 in, 3 out]
  n155 = Select(t=w23, s=w20, f=w4) -> (s? t:f=w24:string)
  "Chaîne" <- w24
  n156 = Not Equal?(x=w15, y=path "") -> (x != y?=w17:bool)
  n157 = Open/Create/Replace File(file path (use dialog)=w50, error in=w26, operation (0:open)=w32) -> (refnum out=w56:refnum<file>, error out=w58:errorcluster)  [unwired: 3 in, 1 out]
  n158 = case shown="True" w17 {
    tunnel: w32 -> [_ w400]
    tunnel: w15 -> [_ w399]
    tunnel: w26 -> [_ w398]
    tunnel: w24 -> [_ w397]
    tunnel: [errorcluster {"status"=FALSE, "code"=0, "source"=""} ("error out") w396] -> w22
    frame False {
    }
    frame True {
      n159 = Open/Create/Replace File(file path (use dialog)=w399, error in=w398, operation (0:open)=w400) -> (refnum out=w401:refnum<file>, error out=w403:errorcluster)  [unwired: 3 in, 1 out]
      n160 = Write to Text File(file (use dialog)=w401, text=w397, error in=w403) -> (refnum out=w402:refnum<file>, error out=w404:errorcluster)  [unwired: 1 in, 1 out]
      n161 = Close File(refnum=w402, error in=w404) -> (error out=w396:errorcluster)  [unwired: 1 out]
    }
  }
  n162 = Write to Text File(file (use dialog)=w56, text=w24, error in=w58) -> (refnum out=w57:refnum<file>, error out=w59:errorcluster)  [unwired: 1 in, 1 out]
  n163 = Close File(refnum=w57, error in=w59) -> (error out=w21:errorcluster)  [unwired: 1 out]
  n164 = Merge Errors(w21, w22) -> (w19:errorcluster)
  "sortie d'erreur" <- w19
  n165 = Compound Arithmetic op=AND ("Opérateur arithmétique")(w20, invert w19) -> (→"tout bon":bool)
